vi "Delete FID Cmd.vi"(1 "ID":i16) -> (0 "Cmd":string)   [LabVIEW 2020]
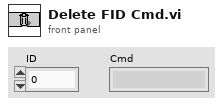
[diagram p1: front panel]
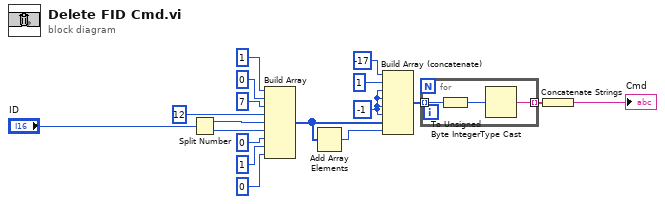
[diagram p0: block diagram]
diagram:
  w6 = i8 -1
  n1 = Split Number(x="ID") -> (hi(x)=w12:u8, lo(x)=w13:u8)
  n2 = Build Array(i8 1, i8 0, i8 7, i8 12, w12, w13, i8 0, i8 1, i8 0) -> (w18:u8[])
  n3 = Add Array Elements(numeric array=w18) -> (sum=w17:u8)
  n4 = Build Array (concatenate)(i8 -17, i8 1, w6, w6, w6, w6, w18, w17) -> (w2:u8[])
  n5 = for {
    tunnel: [w21] -> w1 mode=indexing
    tunnel: w2 -> [w20] mode=indexing
    n6 = To Unsigned Byte Integer(number=w20) -> (unsigned 8bit integer=w19:u8)
    n7 = Type Cast(x=w19) -> (*(type *) &x=w21:string)  [unwired: 1 in]
  }
  n8 = Concatenate Strings(w1) -> (→"Cmd":string)
